vi "LC_BESS_Main.vi"() -> ()   [LabVIEW 2016]
doc: "-----------------------------------------------------------------------------------------------------------------------\nCopyright <2019> <The University of Tennessee at Knoxville and the University of Tennessee Research Foundation>\nThis software is released under BSD-3 a\nhttps://opensource.org/licenses/BSD-3-Clause \nAdditional license options available at https://utrf.tennessee.edu/industry/sample-agreements/\n-----------------------------------------------------------------------------------------------------------------------\n\n\nMain function for BESS LC.\nInclude LC part of resynchronization"
uses:
  LabVIEW Data/MathScriptVIs/MCStatic_36913153632_137dbbc8b62ff179ad17ce13afb809c8.vi
  <instcachedir>/0/MCStatic_36913153632_137dbbc8b62ff179ad17ce13afb809c8_7337D6D141B744C0ACEB8CFFCA4DAD86.lvgen/MCStatic_36913153632_137dbbc8b62ff179ad17ce13afb809c8_7337D6D141B744C0ACEB8CFFCA4DAD86_000.vi
  <vilib>/imath/engines/lvmath2/RunTimeEngine/BuiltInFunctions/abs/NIMS_abs(unsigned).vi
  <instcachedir>/0/NIMS_abs(unsigned)_CB0E2CC90712458C87FBF103B22FBEA1.lvgen/NIMS_abs(unsigned)_CB0E2CC90712458C87FBF103B22FBEA1_002.vi
  <vilib>/imath/engines/lvmath2/RunTimeEngine/NodeEndStatement/NIMS_NodeEndStatement_Output.vi
  <instcachedir>/0/NIMS_NodeEndStatement_Output_53EC0D466D134D7ABD903AC30B43404B.lvgen/NIMS_NodeEndStatement_Output_53EC0D466D134D7ABD903AC30B43404B_001.vi
  <vilib>/imath/engines/lvmath2/RunTimeEngine/ErrorHandling/NIMS_Finalize Error.vi
  LC_BESS_global.vi
  <vilib>/ErrorRing/Error Ring.xnode
  PIcontroller.m
  Communication/DNP3 communication files/Outstation Communication Files/DNP3_Outstation_Template.lvlib
panel:
  out "Waveform Chart":dbl[][](graph)=[[-0.0, 0.25, 0.0]]
  in  "BESS_Active_Power_Cmd 2":fxp<+/-,64,32>=0.25
  in  "Network Settings 1":T1={"port (20000)"=18000, "Master IP"="48.26.87.212", "Master Address"=12345, "Outstation Address "=54321, " update rate"=50}
  in  "DNP3 DataMap 1":T2={"Binary Output Points"=1, "Binary Input Points"=0, "Analog Output Points"=7, "Analog Input Points"=6}
  in  "Settings Cluster":T3={"Default Variation:Analog Input Event (OBJ32)"=1, "Default Variation:Analog Input (OBJ30)"=1, "Default Variation:Binary Input (OBJ01)"=1, "Default Variation:Analog Output (OBJ40)"=4, "Default Variation:Binary Output Event (OBJ11)"=1, "Default Variation:Binary Output (OBJ10)"=1, "Default Variation:Analog Output Event (OBJ42)"=8, "Unsolicited Response Allowed"=FALSE, "Control:Select Timeout (ms)"=0, "Misc:Appl Confirmation Timeout"=0} {"Default Variation:Analog Output Event (OBJ42)" items=["32-bit without Time"=1, "16-bit without Time"=2, "32-bit with Time"=3, "16-bit with Time"=4, "Single-prec without Time"=5, "Double-prec without Time"=6, "Single-prec with Time"=7, "Double-prec with Time"=8]; "Default Variation:Binary Output (OBJ10)" items=["Packed Format"=1, "Output Status with Flags"=2]; "Default Variation:Binary Output Event (OBJ11)" items=["Status without Time"=1, "Status with Time"=2]; "Default Variation:Analog Output (OBJ40)" items=["32-bit with Flag"=1, "16-bit with Flag"=2, "Single-prec with Flag"=3, "Double-prec with Flag"=4]; "Default Variation:Binary Input (OBJ01)" items=["Packed Format"=1, "With Flags"=2]; "Default Variation:Analog Input (OBJ30)" items=["32-bit with Flag"=1, "16-bit with Flag"=2, "32-bit without Flag"=3, "16-bit without Flag"=4, "Single-prec with Flag"=5, "Double-prec with Flag"=6]; "Default Variation:Analog Input Event (OBJ32)" items=["32-bit without Time"=1, "16-bit without Time"=2, "32-bit with Time"=3, "16-bit with Time"=4, "Single-prec without Time"=5, "Double-prec without Time"=6, "Single-prec with Time"=7, "Double-prec with Time"=8]}
  out "MS POLLING? IND":bool=TRUE
  out "OS SETTINGS CHANGED":bool
  in  "ENABLE OS":bool=TRUE
  in  "RESET OS":bool caption="Reset Outstation"
  out "OS SubVI Iterations":i16=8123
  out "MGCC_to_BESS":dbl[](array[numeric])=[1.0, 0.0, 0.0, 0.0, 0.0, 0.0, 0.0] format="%#_6f"
  in  "p_mag":dbl=-1.0
  in  "i_mag":dbl=-1.0
  out "Waveform Chart 2":dbl(graph)
  out "BESS_Start_Stop_Cmd":bool
  out "error out 3":errorcluster
  out "error out 2":errorcluster
  out "BESS_Active_Power_Cmd":fxp<+/-,64,32>=0.25
  in  "Enable":bool=TRUE
  in  "p_in":dbl=0.5
  in  "i_in":dbl=0.2
  in  "p_an":dbl=0.2
  in  "i_an":dbl=0.05
  out "error out":errorcluster
  in  "BESS_Start_Stop":bool
  in  "BESS_Rective_Power_Cmd":fxp<+/-,64,32>=-1.0
  out "BESS_F":fxp<+/-,64,32>=59.92425537109375
  out "BESS_P":fxp<+/-,64,32>=0.000335693359375
  out "BESS_Q":fxp<+/-,64,32>=0.0039520263671875
  out "BESS_V":fxp<+/-,64,32>=0.0112762451171875
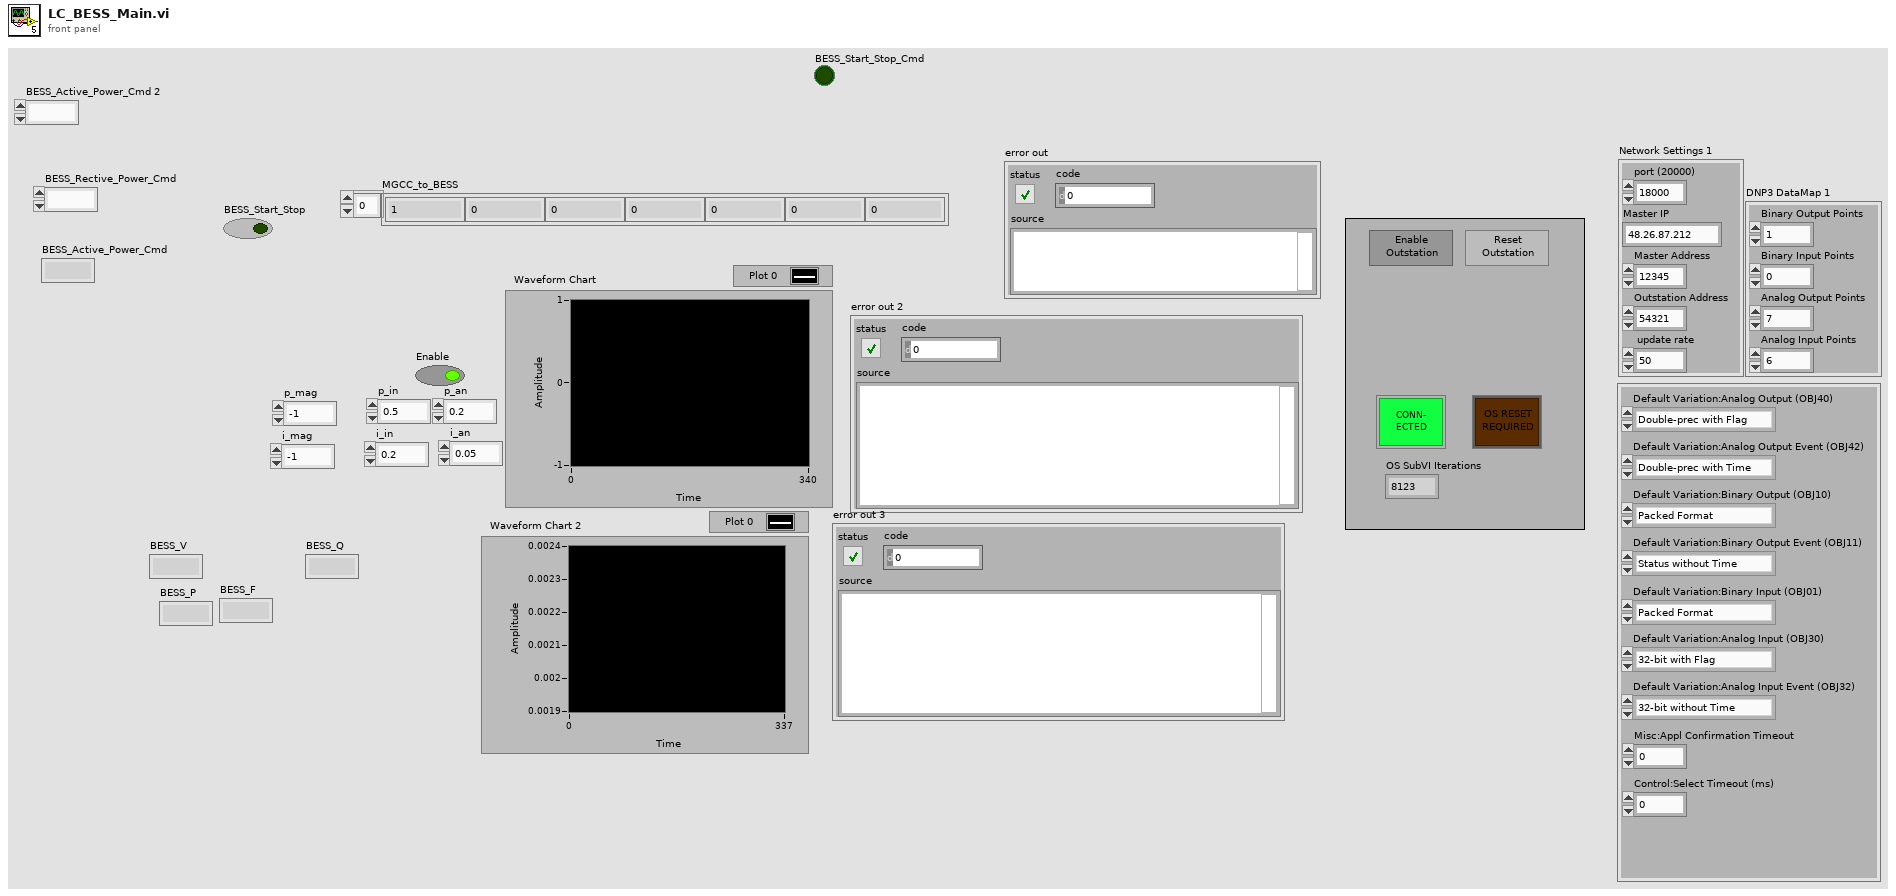
[diagram p1: front panel]
types:
  T1 = cluster{"port (20000)":u16, "Master IP":string, "Master Address":u16, "Outstation Address ":u16, " update rate":u32}
  T2 = cluster{"Binary Output Points":u16, "Binary Input Points":u16, "Analog Output Points":u16, "Analog Input Points":u16}
  T3 = cluster{"Default Variation:Analog Input Event (OBJ32)":u8, "Default Variation:Analog Input (OBJ30)":u8, "Default Variation:Binary Input (OBJ01)":u8, "Default Variation:Analog Output (OBJ40)":u8, "Default Variation:Binary Output Event (OBJ11)":u8, "Default Variation:Binary Output (OBJ10)":u8, "Default Variation:Analog Output Event (OBJ42)":u8, "Unsolicited Response Allowed":bool, "Control:Select Timeout (ms)":u32, "Misc:Appl Confirmation Timeout":u32}
  T4 = cluster{"DNP3 outstation session out":refnum<k21>, "DNP3 outstation out":refnum<k21>, "error out":errorcluster}
  T5 = typedef "NI_Matrix.lvlib/RealMatrix.ctl" = dbl[][]
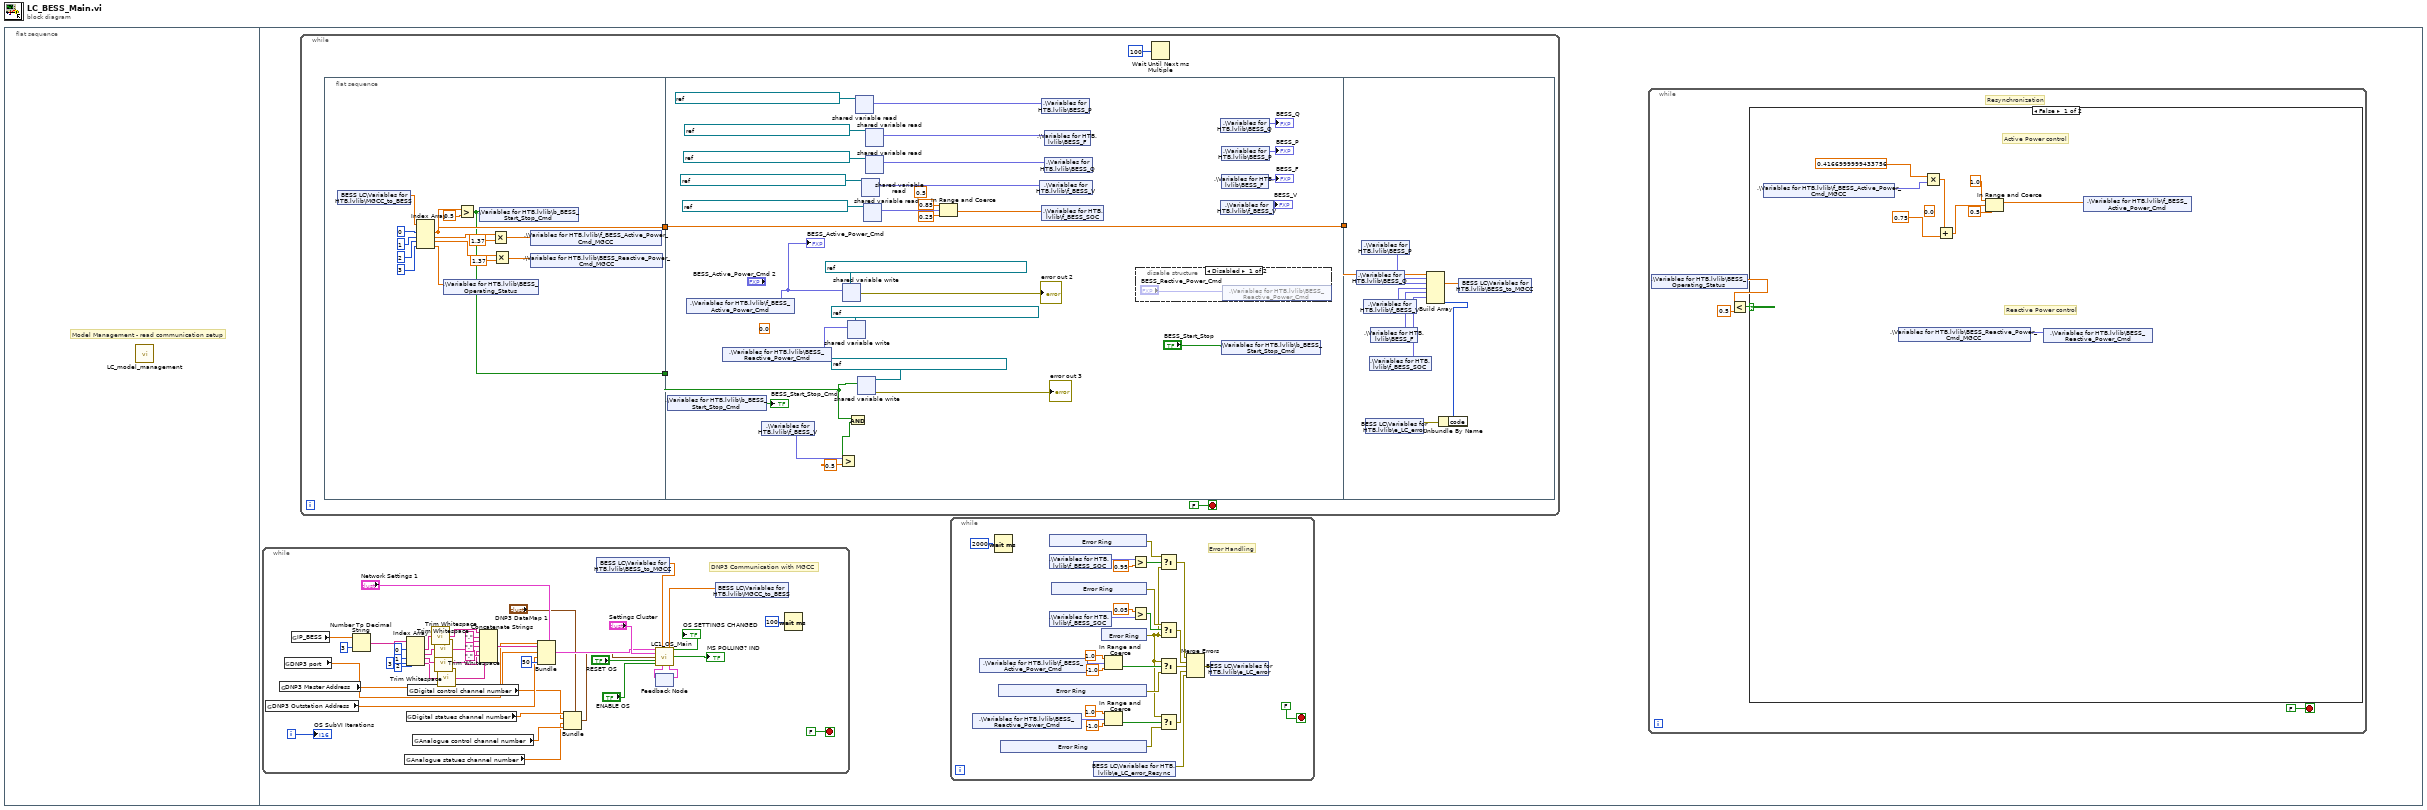
[diagram p0: block diagram]
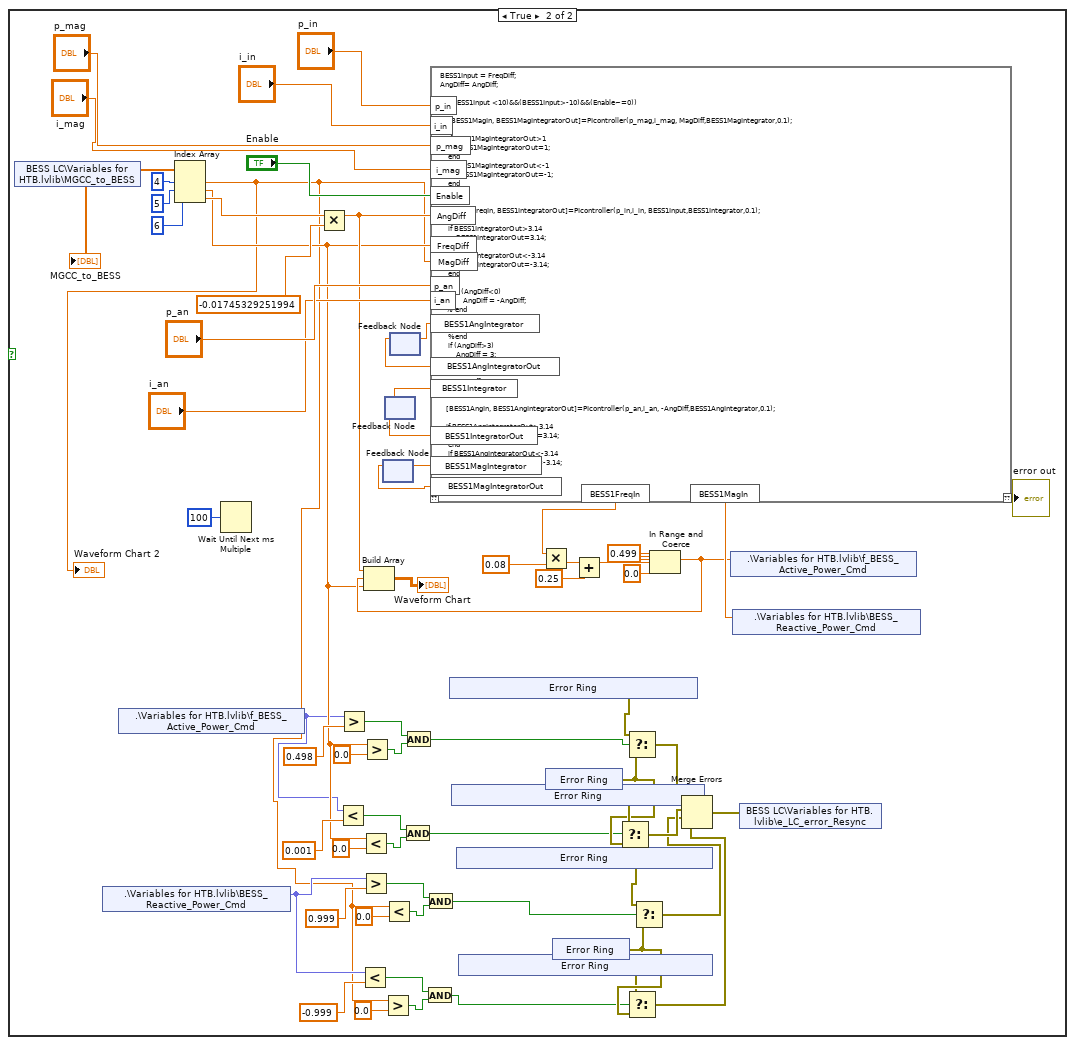
[diagram p2: hidden frame]
diagram:
  n1 = flat-sequence {
    frame #0 {
      # "Model Management - read communication setup"
      n2 = call "LC_model_management.vi"() -> ()  [unwired: 12 in]
    }
    frame #1 {
      n3 = while {
        i -> [w70]
        stop <- FALSE stop-if-true
        # "DNP3 Communication with MGCC"
        n4 = global read "LC_BESS_global.vi" "DNP3 Outstation Address"() -> (w40:dbl)
        n5 = global read "LC_BESS_global.vi" "DNP3 Master Address"() -> (w41:dbl)
        n6 = global read "LC_BESS_global.vi" "DNP3 port"() -> (w42:dbl)
        n7 = global read "LC_BESS_global.vi" "IP_BESS"() -> (w61:dbl[])
        n8 = Number To Decimal String(number=w61, width (-)=i16 3) -> (decimal integer string=w59:string[])
        n9 = global read "LC_BESS_global.vi" "Analogue statues channel number"() -> (w34:dbl)
        n10 = global read "LC_BESS_global.vi" "Digital statues channel number"() -> (w37:dbl)
        n11 = Index Array(array=w59, index #1=0 ("index"), index #2=1 ("index"), index #3=2 ("index"), index #4=3 ("index")) -> (element #1=w51:string, element #2=w49:string, element #3=w47:string, element #4=w45:string)
        n12 = global read "LC_BESS_global.vi" "Digital control channel number"() -> (w36:dbl)
        n13 = global read "LC_BESS_global.vi" "Analogue control channel number"() -> (w35:dbl)
        n14 = call <vilib>:"Trim Whitespace.vi"("string"=w51) -> ("trimmed string"=w50:string)  [unwired: 1 in]
        n15 = call <vilib>:"Trim Whitespace.vi"("string"=w49) -> ("trimmed string"=w48:string)  [unwired: 1 in]
        n16 = call <vilib>:"Trim Whitespace.vi"("string"=w47) -> ("trimmed string"=w46:string)  [unwired: 1 in]
        n17 = call <vilib>:"Trim Whitespace.vi"("string"=w45) -> ("trimmed string"=w44:string)  [unwired: 1 in]
        n18 = Concatenate Strings(w50, "." ("string"), w48, "." ("string"), w46, "." ("string"), w44) -> (w43:string)
        n19 = Bundle(cluster="Network Settings 1", "port (20000)"=w42, "Master IP"=w43, "Master Address"=w41, "Outstation Address"=w40, "update rate"=u32 50) -> (w39:T1)
        n20 = Bundle(cluster="DNP3 DataMap 1", "Binary Output Points"=w37, "Binary Input Points"=w36, "Analog Output Points"=w34, "Analog Input Points"=w35) -> (w33:T2)
        n21 = shared-variable "BESS LC\\Variables for HTB.lvlib\\BESS_to_MGCC"() -> (w64:dbl[])  [unwired: 1 in, 1 out]
        n22 = feedback #1() -> (w68:T4)  [unwired: 1 in]
        n23 = call "LC1_OS_Main.vi"("Network Settings 1"=w39, "Analog Input"=w64, "Settings Cluster"="Settings Cluster", "DNP3 DataMap 1"=w33, "OS_Reset"="RESET OS", "OS_Enable"="ENABLE OS", "DNP3 Session Input"=w68) -> ("Analog Output"=w65:dbl[], "OS_DNP3_Settings_Changed"=→"OS SETTINGS CHANGED":bool, "Connected?"=→"MS POLLING? IND":bool, "DNP3 Session"=w69:T4)  [unwired: 5 in]
        n24 = feedback-in #1(w69) -> ()
        n25 = shared-variable "BESS LC\\Variables for HTB.lvlib\\MGCC_to_BESS"(w65) -> ()  [unwired: 1 in, 1 out]
        n26 = Wait (ms)(milliseconds to wait=u32 100) -> ()  [unwired: 1 out]
        "OS SubVI Iterations" <- w70
      }
      n27 = while {
        stop <- FALSE stop-if-true
        n28 = flat-sequence {
          tunnel: [w629] -> w616
          tunnel: [w626] -> w615
          tunnel: [w652] -> w617
          tunnel: w616 -> [w652]
          tunnel: w615 -> [w648]
          tunnel: w617 -> [w669]
          frame #0 {
            n29 = shared-variable "BESS LC\\Variables for HTB.lvlib\\MGCC_to_BESS"() -> (w634:dbl[])  [unwired: 1 in, 1 out]
            n30 = Index Array(array=w634, index #1=0 ("index"), index #2=1 ("index"), index #3=2 ("index"), index #4=3 ("index")) -> (element #1=w629:dbl, element #2=w625:dbl, element #3=w621:dbl, element #4=w627:dbl)
            n31 = shared-variable ".\\Variables for HTB.lvlib\\BESS_Operating_Status"(w627) -> ()  [unwired: 1 in, 1 out]
            n32 = Greater?(x=w629, y=0.5) -> (0:w626:bool)
            n33 = shared-variable ".\\Variables for HTB.lvlib\\b_BESS_Start_Stop_Cmd"(w626) -> ()  [unwired: 1 in, 1 out]
            n34 = Multiply(x=w625, y=1.37) -> (x*y=w624:dbl)
            n35 = Multiply(x=w621, y=1.37) -> (x*y=w622:dbl)
            n36 = shared-variable ".\\Variables for HTB.lvlib\\f_BESS_Active_Power_Cmd_MGCC"(w624) -> ()  [unwired: 1 in, 1 out]
            n37 = shared-variable ".\\Variables for HTB.lvlib\\BESS_Reactive_Power_Cmd_MGCC"(w622) -> ()  [unwired: 1 in, 1 out]
          }
          frame #1 {
            (unwired) 0.5
            (unwired) 0.0 ("lower limit")
            n38 = shared-variable ".\\Variables for HTB.lvlib\\b_BESS_Start_Stop_Cmd"() -> (→"BESS_Start_Stop_Cmd":bool)  [unwired: 1 in, 1 out]
            n39 = shared-variable ".\\Variables for HTB.lvlib\\f_BESS_Active_Power_Cmd"() -> (w637:fxp<+/-,64,32>)  [unwired: 1 in, 1 out]
            "BESS_Active_Power_Cmd" <- w637
            n40 = shared-variable ".\\Variables for HTB.lvlib\\BESS_Reactive_Power_Cmd"() -> (w636:fxp<+/-,64,32>)  [unwired: 1 in, 1 out]
            n41 = shared-variable ".\\Variables for HTB.lvlib\\f_BESS_V"() -> (w644:fxp<+/-,64,32>)  [unwired: 1 in, 1 out]
            n42 = Greater?(x=w644, y=0.5) -> (0:w649:bool)
            n43 = shared-variable-write(refnum<k21> "ni.var.psp://cepd00622/Variables from Host/L1 Active Power" ("shared variable refnum in"), w637) -> (→"error out 2":errorcluster)  [unwired: 1 in, 1 out]
            n44 = shared-variable-write(refnum<k21> "ni.var.psp://cepd00622/Variables from Host/L1 Reactive Power" ("shared variable refnum in"), w636) -> ()  [unwired: 1 in, 2 out]
            n45 = And(x=w648, y=w649) -> ()  [unwired: 1 out]
            n46 = shared-variable-read(refnum<k21> "ni.var.psp://cepd00622/Variables from Host/L1 P" ("shared variable refnum in")) -> (w655:fxp<+/-,64,32>)  [unwired: 1 in, 2 out]
            n47 = shared-variable-write(refnum<k21> "ni.var.psp://cepd00622/Variables from Host/L1 Start" ("shared variable refnum in"), w648) -> (→"error out 3":errorcluster)  [unwired: 1 in, 1 out]
            n48 = shared-variable-read(refnum<k21> "ni.var.psp://cepd00622/Variables from Host/L1 V" ("shared variable refnum in")) -> (w660:fxp<+/-,64,32>)  [unwired: 1 in, 2 out]
            n49 = shared-variable-read(refnum<k21> "ni.var.psp://cepd00622/Variables from Host/L8 V" ("shared variable refnum in")) -> (w638:fxp<+/-,64,32>)  [unwired: 1 in, 2 out]
            n50 = shared-variable-read(refnum<k21> "ni.var.psp://cepd00622/Variables from Host/L1 F" ("shared variable refnum in")) -> (w643:fxp<+/-,64,32>)  [unwired: 1 in, 2 out]
            n51 = shared-variable-read(refnum<k21> "ni.var.psp://cepd00622/Variables from Host/L1 Q" ("shared variable refnum in")) -> (w657:fxp<+/-,64,32>)  [unwired: 1 in, 2 out]
            n52 = In Range and Coerce(upper limit=0.85, x=w638, lower limit=0.25) -> (coerced(x)=w635:dbl)  [unwired: 1 out]
            n53 = shared-variable ".\\Variables for HTB.lvlib\\f_BESS_V"(w660) -> ()  [unwired: 1 in, 1 out]
            n54 = shared-variable ".\\Variables for HTB.lvlib\\BESS_P"(w655) -> ()  [unwired: 1 in, 1 out]
            n55 = shared-variable ".\\Variables for HTB.lvlib\\f_BESS_SOC"(w635) -> ()  [unwired: 1 in, 1 out]
            n56 = shared-variable ".\\Variables for HTB.lvlib\\BESS_F"(w643) -> ()  [unwired: 1 in, 1 out]
            n57 = shared-variable ".\\Variables for HTB.lvlib\\BESS_Q"(w657) -> ()  [unwired: 1 in, 1 out]
            n58 = disable-structure shown="Disabled" {
              frame Disabled {
                n59 = shared-variable ".\\Variables for HTB.lvlib\\BESS_Reactive_Power_Cmd"("BESS_Rective_Power_Cmd") -> ()  [unwired: 1 in, 1 out]
              }
              frame Enabled {
              }
            }
            n60 = shared-variable ".\\Variables for HTB.lvlib\\BESS_Q"() -> (→"BESS_Q":fxp<+/-,64,32>)  [unwired: 1 in, 1 out]
            n61 = shared-variable ".\\Variables for HTB.lvlib\\f_BESS_V"() -> (→"BESS_V":fxp<+/-,64,32>)  [unwired: 1 in, 1 out]
            n62 = shared-variable ".\\Variables for HTB.lvlib\\BESS_P"() -> (→"BESS_P":fxp<+/-,64,32>)  [unwired: 1 in, 1 out]
            n63 = shared-variable ".\\Variables for HTB.lvlib\\BESS_F"() -> (→"BESS_F":fxp<+/-,64,32>)  [unwired: 1 in, 1 out]
            n64 = shared-variable ".\\Variables for HTB.lvlib\\b_BESS_Start_Stop_Cmd"("BESS_Start_Stop") -> ()  [unwired: 1 in, 1 out]
          }
          frame #2 {
            n65 = shared-variable ".\\Variables for HTB.lvlib\\BESS_Q"() -> (w674:fxp<+/-,64,32>)  [unwired: 1 in, 1 out]
            n66 = shared-variable ".\\Variables for HTB.lvlib\\BESS_P"() -> (w675:fxp<+/-,64,32>)  [unwired: 1 in, 1 out]
            n67 = shared-variable ".\\Variables for HTB.lvlib\\f_BESS_V"() -> (w673:fxp<+/-,64,32>)  [unwired: 1 in, 1 out]
            n68 = shared-variable "BESS LC\\Variables for HTB.lvlib\\e_LC_error"() -> (w668:errorcluster)  [unwired: 1 in, 1 out]
            n69 = shared-variable ".\\Variables for HTB.lvlib\\f_BESS_SOC"() -> (w670:fxp<+/-,64,32>)  [unwired: 1 in, 1 out]
            n70 = shared-variable ".\\Variables for HTB.lvlib\\BESS_F"() -> (w672:fxp<+/-,64,32>)  [unwired: 1 in, 1 out]
            n71 = Unbundle By Name(w668) -> ("code"=w667:i32)
            n72 = Build Array(w669, w675, w674, w673, w672, w670, w667) -> (w671:dbl[])
            n73 = shared-variable "BESS LC\\Variables for HTB.lvlib\\BESS_to_MGCC"(w671) -> ()  [unwired: 1 in, 1 out]
          }
        }
        n74 = Wait Until Next ms Multiple(millisecond multiple=u32 100 ("milliseconds to wait")) -> ()  [unwired: 1 out]
      }
      n75 = while {
        stop <- FALSE stop-if-true
        # "Error Handling"
        n76 = shared-variable ".\\Variables for HTB.lvlib\\BESS_Reactive_Power_Cmd"() -> (w2:fxp<+/-,64,32>)  [unwired: 1 in, 1 out]
        n77 = shared-variable ".\\Variables for HTB.lvlib\\f_BESS_Active_Power_Cmd"() -> (w12:fxp<+/-,64,32>)  [unwired: 1 in, 1 out]
        n78 = Wait (ms)(milliseconds to wait=u32 2000) -> ()  [unwired: 1 out]
        n79 = xnode "Error Ring"() -> ("error out"=w10:errorcluster)
        n80 = xnode "Error Ring"() -> ("error out"=w5:errorcluster)
        n81 = xnode "Error Ring"() -> ("error out"=w21:errorcluster)
        n82 = shared-variable ".\\Variables for HTB.lvlib\\f_BESS_SOC"() -> (w25:fxp<+/-,64,32>)  [unwired: 1 in, 1 out]
        n83 = shared-variable ".\\Variables for HTB.lvlib\\f_BESS_SOC"() -> (w18:fxp<+/-,64,32>)  [unwired: 1 in, 1 out]
        n84 = xnode "Error Ring"() -> ("error out"=w16:errorcluster)
        n85 = shared-variable "BESS LC\\Variables for HTB.lvlib\\e_LC_error_Resync"() -> (w1:errorcluster)  [unwired: 1 in, 1 out]
        n86 = xnode "Error Ring"() -> ("error out"=w4:errorcluster)
        n87 = In Range and Coerce(upper limit=1.0, x=w12, lower limit=-1.0) -> (In Range?=w11:bool)  [unwired: 1 out]
        n88 = In Range and Coerce(upper limit=1.0, x=w2, lower limit=-1.0) -> (In Range?=w8:bool)  [unwired: 1 out]
        n89 = Greater?(x=w25, y=0.95 ("upper limit")) -> (0:w22:bool)
        n90 = Greater?(x=0.05 ("lower limit"), y=w18) -> (0:w17:bool)
        n91 = Select(t=w21, s=w22, f=w4) -> (s? t:f=w20:errorcluster)
        n92 = Select(t=w16, s=w17, f=w4) -> (s? t:f=w15:errorcluster)
        n93 = Select(t=w4, s=w11, f=w10) -> (s? t:f=w9:errorcluster)
        n94 = Select(t=w4, s=w8, f=w5) -> (s? t:f=w3:errorcluster)
        n95 = Merge Errors(w20, w15, w9, w3, w1) -> (w23:errorcluster)
        n96 = shared-variable "BESS LC\\Variables for HTB.lvlib\\e_LC_error"(w23) -> ()  [unwired: 1 in, 1 out]
      }
      n97 = while {
        stop <- FALSE stop-if-true
        # "Resynchronization"
        n98 = shared-variable ".\\Variables for HTB.lvlib\\BESS_Operating_Status"() -> (w78:dbl)  [unwired: 1 in, 1 out]
        n99 = Less?(x=w78, y=0.5) -> (x < y?=w76:bool)
        n100 = case shown="False" w76 {
          frame False {
            (unwired) 0.0 ("x")
            # "Reactive Power control"
            # "Active Power control"
            n101 = shared-variable ".\\Variables for HTB.lvlib\\f_BESS_Active_Power_Cmd_MGCC"() -> (w84:fxp<+/-,64,32>)  [unwired: 1 in, 1 out]
            n102 = shared-variable ".\\Variables for HTB.lvlib\\BESS_Reactive_Power_Cmd_MGCC"() -> (w82:fxp<+/-,64,32>)  [unwired: 1 in, 1 out]
            n103 = Multiply(x=0.4166999999433756 ("BESS_Active_Power_Cmd"), y=w84) -> (x*y=w81:dbl)
            n104 = Add(x=w81, y=0.75 ("BESS_Active_Power_Cmd")) -> (x+y=w86:dbl)
            n105 = In Range and Coerce(upper limit=1.0, x=w86, lower limit=0.5) -> (coerced(x)=w80:dbl)  [unwired: 1 out]
            n106 = shared-variable ".\\Variables for HTB.lvlib\\BESS_Reactive_Power_Cmd"(w82) -> ()  [unwired: 1 in, 1 out]
            n107 = shared-variable ".\\Variables for HTB.lvlib\\f_BESS_Active_Power_Cmd"(w80) -> ()  [unwired: 1 in, 1 out]
          }
          frame True {
            n108 = shared-variable "BESS LC\\Variables for HTB.lvlib\\MGCC_to_BESS"() -> (w137:dbl[])  [unwired: 1 in, 1 out]
            "MGCC_to_BESS" <- w137
            n109 = shared-variable ".\\Variables for HTB.lvlib\\BESS_Reactive_Power_Cmd"() -> (w97:fxp<+/-,64,32>)  [unwired: 1 in, 1 out]
            n110 = shared-variable ".\\Variables for HTB.lvlib\\f_BESS_Active_Power_Cmd"() -> (w98:fxp<+/-,64,32>)  [unwired: 1 in, 1 out]
            n111 = Index Array(array=w137, index #1=4 ("index"), index #2=5 ("index"), index #3=6 ("index")) -> (element #1=w96:dbl, element #2=w108:dbl, element #3=w133:dbl)
            "Waveform Chart 2" <- w96
            n112 = Wait Until Next ms Multiple(millisecond multiple=u32 100) -> ()  [unwired: 1 out]
            n113 = Multiply(x=w133, y=-0.01745329251994) -> (x*y=w125:dbl)
            n114 = Less?(x=w98, y=0.001 ("upper limit")) -> (x < y?=w110:bool)
            n115 = Greater?(x=w98, y=0.498 ("upper limit")) -> (0:w122:bool)
            n116 = Less?(x=w97, y=-0.999 ("upper limit")) -> (x < y?=w105:bool)
            n117 = Less?(x=w108, y=0.0) -> (x < y?=w112:bool)
            n118 = Greater?(x=w97, y=0.999 ("upper limit")) -> (0:w100:bool)
            n119 = Greater?(x=w108, y=0.0) -> (0:w120:bool)
            n120 = feedback #2() -> (w128:dbl)  [unwired: 1 in]
            n121 = Greater?(x=w96, y=0.0) -> (0:w103:bool)
            n122 = Less?(x=w96, y=0.0) -> (x < y?=w102:bool)
            n123 = feedback #3() -> (w155:dbl)  [unwired: 1 in]
            n124 = feedback #4() -> (w152:dbl)  [unwired: 1 in]
            n125 = And(x=w110, y=w112) -> (x .and. y?=w107:bool)
            n126 = And(x=w122, y=w120) -> (x .and. y?=w113:bool)
            n127 = And(x=w105, y=w103) -> (x .and. y?=w89:bool)
            n128 = And(x=w100, y=w102) -> (x .and. y?=w90:bool)
            n129 = mathscript code="BESS1Input = FreqDiff;\nAngDiff= AngDiff;\n\nif ((BESS1Input <10)&&(BESS1Input>-10)&&(Enable~=0))\n\n    [BESS1MagIn, BESS1MagIntegratorOut]=PIcontroller(p_mag,i_mag, MagDiff,BESS1MagIntegrator,0.1);\n   \n    if BESS1MagIntegratorOut>1\n        BESS1MagIntegratorOut=1;\n    end\n    if BESS1MagIntegratorOut<-1\n        BESS1MagIntegratorOut=-1;\n    end\n\n\n    [BESS1FreqIn, BESS1IntegratorOut]=PIcontroller(p_in,i_in, BESS1Input,BESS1Integrator,0.1);\n   \n    if BESS1IntegratorOut>3.14\n        BESS1IntegratorOut=3.14;\n    end\n    if BESS1IntegratorOut<-3.14\n        BESS1IntegratorOut=-3.14;\n    end\n\n%    if (AngDiff<0)\n %       AngDiff = -AngDiff;\n   % end \n    %if (AngDiff> 5)\n     %   AngDiff = 0;\n    %end \n    if (AngDiff>3)\n        AngDiff = 3;\n    end \n    if (AngDiff<-3)\n        AngDiff = -3;\n    end \n\n   [BESS1AngIn, BESS1AngIntegratorOut]=PIcontroller(p_an,i_an, -AngDiff,BESS1AngIntegrator,0.1);\n\n   if BESS1AngIntegratorOut>3.14\n        BESS1AngIntegratorOut=3.14;\n    end\n    if BESS1AngIntegratorOut<-3.14\n        BESS1AngIntegratorOut=-3.14;\n    end\n    \n    if abs(FreqDiff<0.2)\n        BESS1FreqIn = BESS1FreqIn + BESS1AngIn;\n    else\n        BESS1AngIntegratorOut = 0;\n    end\n    if (BESS1FreqIn > 3.14) \n          BESS1FreqIn = 3.14;\n    end\n    if (BESS1FreqIn < -3.14) \n          BESS1FreqIn = -3.14;\n    end\n\n    if (AngDiff ==0)&&(FreqDiff == 0) && (MagDiff== 0)\n        BESS1FreqIn = 0;\n        BESS1MagIn = 0;\n        BESS1IntegratorOut = 0;\n        BESS1MagIntegratorOut = 0;\n        BESS1AngIntegratorOut = 0;\n    end\n\nelse\nBESS1FreqIn = 0;\nBESS1MagIn = 0;\nBESS1IntegratorOut = 0;\nBESS1MagIntegratorOut = 0;\nBESS1AngIntegratorOut = 0;\nend"("AngDiff"=w125, "BESS1Integrator"=w155, "FreqDiff"=w108, "BESS1AngIntegrator"=w152, "Enable"="Enable", "p_in"="p_in", "i_in"="i_in", "p_an"="p_an", "i_an"="i_an", "p_mag"="p_mag", "i_mag"="i_mag", "BESS1MagIntegrator"=w128, "MagDiff"=w96) -> ("??"=→"error out":errorcluster, "BESS1IntegratorOut"=w154:dbl, "BESS1FreqIn"=w129:dbl, "BESS1AngIntegratorOut"=w153:dbl, "BESS1MagIntegratorOut"=w130:dbl, "BESS1MagIn"=w127:dbl)  [unwired: 1 in]
            n130 = feedback-in #2(w130) -> ()
            n131 = feedback-in #3(w154) -> ()
            n132 = feedback-in #4(w153) -> ()
            n133 = xnode "Error Ring"() -> ("error out"=w118:errorcluster)
            n134 = xnode "Error Ring"() -> ("error out"=w116:errorcluster)
            n135 = xnode "Error Ring"() -> ("error out"=w93:errorcluster)
            n136 = xnode "Error Ring"() -> ("error out"=w94:errorcluster)
            n137 = Multiply(x=w129, y=0.08 ("upper limit")) -> (x*y=w141:dbl)
            n138 = xnode "Error Ring"() -> ("error out"=w114:errorcluster)
            n139 = xnode "Error Ring"() -> ("error out"=w95:errorcluster)
            n140 = Add(x=w141, y=0.25) -> (x+y=w139:dbl)
            n141 = Select(t=w116, s=w107, f=w114) -> (s? t:f=w115:errorcluster)
            n142 = Select(t=w118, s=w113, f=w114) -> (s? t:f=w117:errorcluster)
            n143 = Select(t=w94, s=w89, f=w95) -> (s? t:f=w91:errorcluster)
            n144 = Select(t=w93, s=w90, f=w95) -> (s? t:f=w92:errorcluster)
            n145 = In Range and Coerce(upper limit=0.499, x=w139, lower limit=0.0) -> (coerced(x)=w124:dbl)  [unwired: 1 out]
            n146 = Build Array(w125, w124, w108) -> (→"Waveform Chart":T5)
            n147 = Merge Errors(w117, w115, w92, w91) -> (w119:errorcluster)
            n148 = shared-variable ".\\Variables for HTB.lvlib\\f_BESS_Active_Power_Cmd"(w124) -> ()  [unwired: 1 in, 1 out]
            n149 = shared-variable ".\\Variables for HTB.lvlib\\BESS_Reactive_Power_Cmd"(w127) -> ()  [unwired: 1 in, 1 out]
            n150 = shared-variable "BESS LC\\Variables for HTB.lvlib\\e_LC_error_Resync"(w119) -> ()  [unwired: 1 in, 1 out]
          }
        }
      }
    }
  }
